vi "Import - Rx Packets.vi"(7 "Rx Packets":T1 {"Rx Packet Data"."Endianness" items=["big-endian"=0, "little-endian"=2]}, 8 "error in (no error)":errorcluster, 11 "Device Item Ref in":T8 format="%.0x") -> (0 "error out":errorcluster)   [LabVIEW 2016, in "UDP-Custom-Device System Explorer.lvlib"]
uses:
  UDP-Custom-Device System Explorer.lvlib
  <vilib>/NI Veristand/Custom Device API/Custom Device Item Ref.ctl
  Types/XML - New/ImpExp - Rx Packets Data.ctl
  <vilib>/NI Veristand/Custom Device API/Custom Device Item Info.ctl
  Types/XML - New/ImpExp - Rx Packet Data.ctl
  Shared/Types/Shared - Channel Data Type.ctl
  Shared/Types/Shared - Buffered.PacketInfo.ctl
  Shared/Types/Shared - Pointer Encoding.ctl
  Shared/Types/Shared - New Data Options.ctl
  Property Accessors/Shared Section Accessors.lvlib
  <vilib>/NI VeriStand/Custom Device API/Custom Device API.lvlib
  Shared/UDP-Custom-Device Shared.lvlib
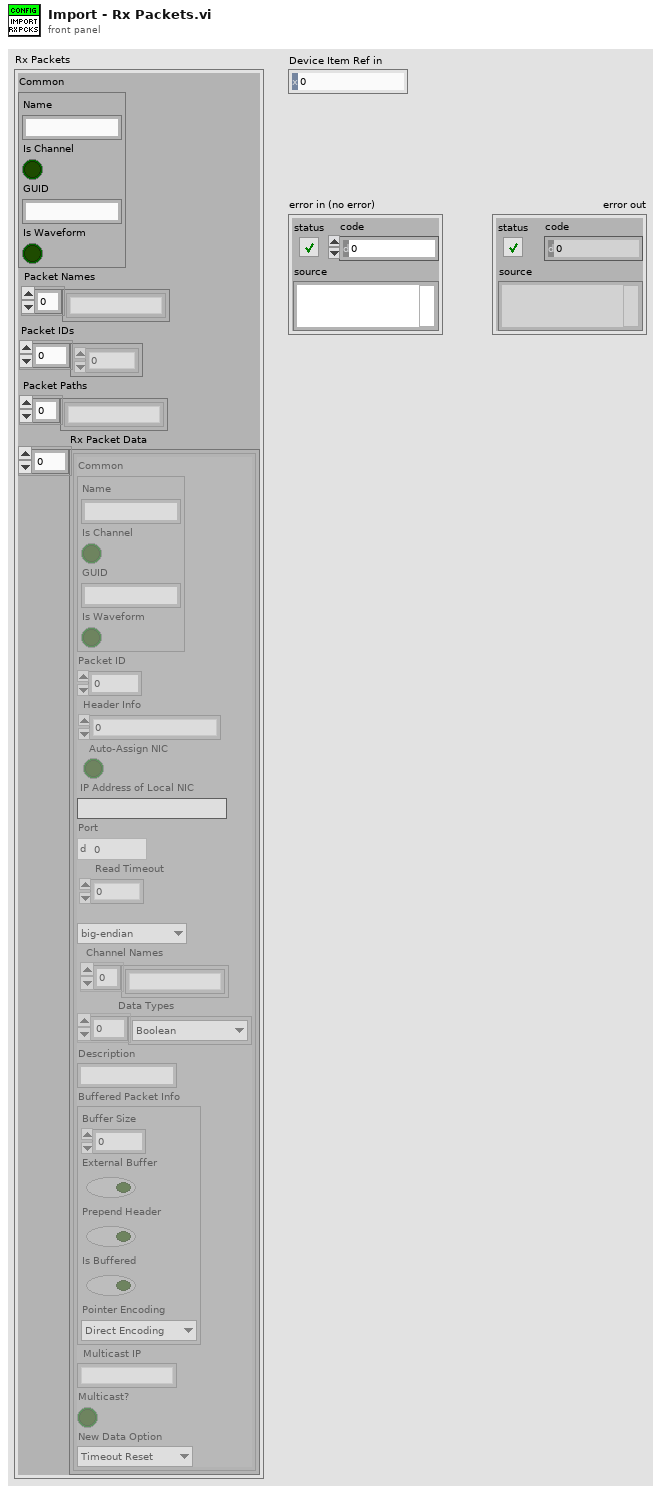
[diagram p1: front panel]
types:
  T1 = typedef "UDP-Custom-Device System Explorer.lvlib/ImpExp - Rx Packets Data.ctl" = cluster{"Common":T2, "Packet Names":string[], "Packet IDs":i32[], "Packet Paths":string[], "Rx Packet Data":T3[]}
  T2 = typedef "Custom Device API.lvlib/Custom Device Item Info.ctl" = cluster{"Name":string, "Is Channel":bool, "GUID":string, "Is Waveform":bool}
  T3 = typedef "UDP-Custom-Device System Explorer.lvlib/ImpExp - Rx Packet Data.ctl" = cluster{"Common":T2, "Packet ID":i32, "Header Info":u32, "Auto-Assign NIC":bool, "IP Address of Local NIC":string, "Port":u16, "Read Timeout":i32, "Endianness":u16, "Channel Names":string[], "Data Types":T4[], "Description":string, "Buffered Packet Info":T5, "Multicast IP":string, "Multicast?":bool, "New Data Option":T7}
  T4 = typedef "UDP-Custom-Device Shared.lvlib/Shared - Channel Data Type.ctl" = enum16{"Boolean", "Single", "Double", "I8", "I16", "I32", "I64", "U8", "U16", "U32", "U64"}
  T5 = typedef "UDP-Custom-Device Shared.lvlib/Shared - Buffered.PacketInfo.ctl" = cluster{"Buffer Size":i32, "External Buffer":bool, "Prepend Header":bool, "Is Buffered":bool, "Pointer Encoding":T6}
  T6 = typedef "UDP-Custom-Device Shared.lvlib/Shared - Pointer Encoding.ctl" = enum16{"Direct Encoding", "Conversion Encoding"}
  T7 = typedef "UDP-Custom-Device Shared.lvlib/Shared - New Data Options.ctl" = enum16{"Timeout Reset", "Counter"}
  T8 = typedef "Custom Device API.lvlib/Custom Device Item Ref.ctl" = u64
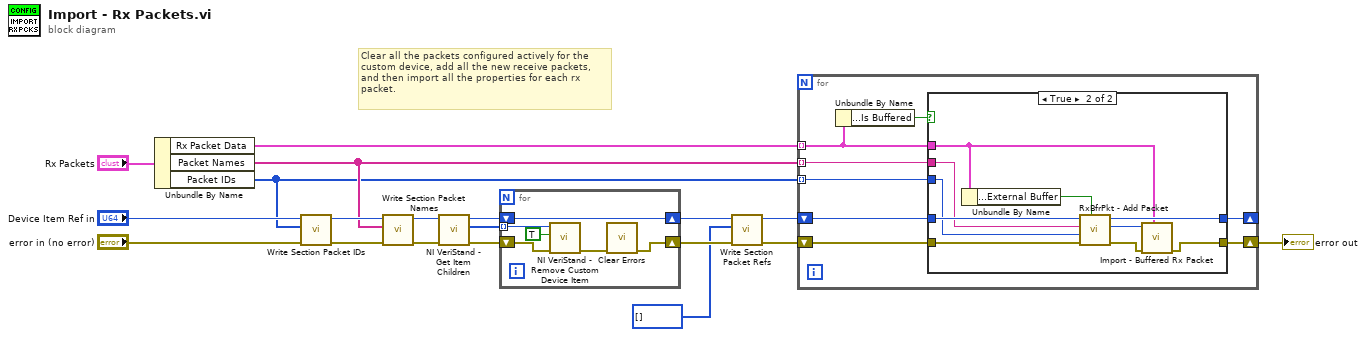
[diagram p0: block diagram]
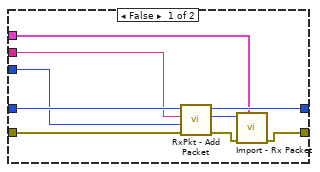
[diagram p2: hidden frame]
diagram:
  # "Clear all the packets configured actively for the\ncustom device, add all the new receive packets,\nand then import all the properties for each rx\npacket."
  n1 = Unbundle By Name("Rx Packets") -> ("Rx Packet Data"=w9:T3[], "Packet Names"=w8:string[], "Packet IDs"=w7:i32[])
  n2 = call "Write Section Packet IDs.vi"("error in (no error)"="error in (no error)", "Packet IDs"=w7, "Node Ptr"="Device Item Ref in") -> ("error out"=w15:errorcluster, "Node Ptr out"=w16:T8)  [unwired: 7 in]
  n3 = call "Write Section Packet Names.vi"("error in (no error)"=w15, "Packet Names"=w8, "Node Ptr"=w16) -> ("error out"=w10:errorcluster, "Node Ptr out"=w11:T8)  [unwired: 7 in]
  n4 = call <vilib>:"NI VeriStand - Get Item Children.vi"("error in (no error)"=w10, "Item Ref in"=w11) -> ("error out"=w14:errorcluster, "Child Refs"=w13:T8[], "Item Ref out"=w12:T8)  [unwired: 6 in, 1 out]
  n5 = for {
    shift-right: [w20] -> w3
    shift-left: w14 -> [w25]
    tunnel: w13 -> [w24] mode=indexing
    shift-right: [w23] -> w5
    shift-left: w12 -> [w23]
    n6 = call <vilib>:"NI VeriStand - Remove Custom Device Item.vi"("error in (no error)"=w25, "Force Delete (F)"=TRUE, "Item Ref in"=w24) -> ("error out"=w21:errorcluster)  [unwired: 7 in, 1 out]
    n7 = call <vilib>:"Clear Errors.vi"("error in (no error)"=w21) -> ("error out"=w20:errorcluster)  [unwired: 5 in, 1 out]
  }
  n8 = call "Write Section Packet Refs.vi"("error in (no error)"=w3, "Dependent Node Refs"=T8[] [], "Node Ptr"=w5) -> ("error out"=w2:errorcluster, "Node Ptr out"=w4:T8)  [unwired: 7 in]
  n9 = for {
    tunnel: w9 -> [w27] mode=indexing
    tunnel: w8 -> [w31] mode=indexing
    tunnel: w7 -> [w30] mode=indexing
    shift-right: [w33] -> w6
    shift-left: w2 -> [w29]
    shift-right: [w28] -> _
    shift-left: w4 -> [w32]
    n10 = Unbundle By Name(w27) -> ("Buffered Packet Info.Is Buffered"=w26:bool)
    n11 = case shown="True" w26 {
      tunnel: [w42 w45] -> w33
      tunnel: w32 -> [w41 w52]
      tunnel: w31 -> [w40 w50]
      tunnel: w30 -> [w39 w49]
      tunnel: w29 -> [w38 w51]
      tunnel: [w35 w48] -> w28
      tunnel: w27 -> [w34 w44]
      frame False {
        n12 = call "RxPkt - Add Packet.vi"("error in (no error)"=w38, "New Packet ID"=w39, "New Packet Name"=w40, "Item Ref in"=w41) -> ("error out"=w37:errorcluster, "New Packet Ref"=w36:T8, "Item Ref Out"=w35:T8)  [unwired: 5 in]
        n13 = call "Import - Rx Packet.vi"("Rx Packet"=w34, "error in (no error)"=w37, "Device Item Ref in"=w36) -> ("error out"=w42:errorcluster)  [unwired: 8 in]
      }
      frame True {
        n14 = Unbundle By Name(w44) -> ("Buffered Packet Info.External Buffer"=w43:bool)
        n15 = call "RxBfrPkt - Add Packet.vi"("Ext Buffer?"=w43, "error in (no error)"=w51, "New Packet ID"=w49, "New Packet Name"=w50, "Item Ref in"=w52) -> ("error out"=w46:errorcluster, "New Packet Ref"=w47:T8, "Item Ref Out"=w48:T8)  [unwired: 4 in]
        n16 = call "Import - Buffered Rx Packet.vi"("Rx Packet"=w44, "error in (no error)"=w46, "Device Item Ref in"=w47) -> ("error out"=w45:errorcluster)  [unwired: 8 in]
      }
    }
  }
  "error out" <- w6
